vi "PicoStatus.vi"(1 "PICO STATUS":u32, 2 "error in":errorcluster, 3 "source":string) -> (0 "error out":errorcluster)   [LabVIEW 2016]
doc: "This VI checks the status value returned by calls to the driver. If the driver returns an error, the status member of the error cluster is set to 'true' and the error code and source are set."
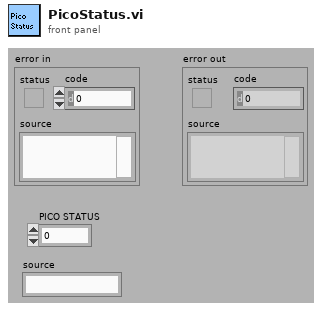
[diagram p1: front panel]
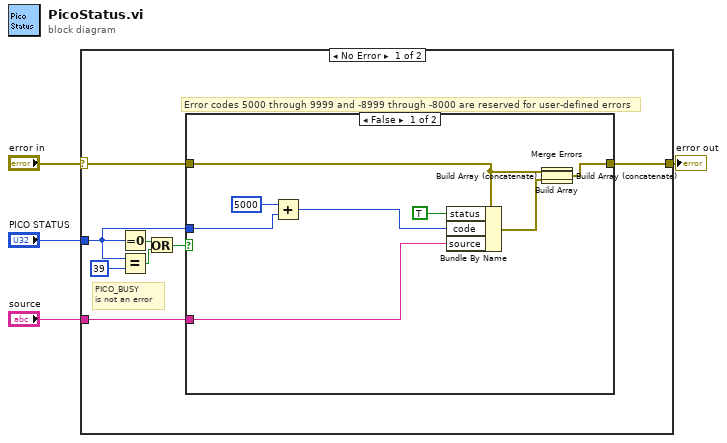
[diagram p0: block diagram]
diagram:
  n1 = case shown="No Error" "error in" {
    selector: "error in" -> [w11 w25]
    tunnel: [w12 w25] -> w4
    tunnel: "PICO STATUS" -> [w6 _]
    tunnel: "source" -> [w10 _]
    frame No Error {
      # "PICO_BUSY \nis not an error"
      # "Error codes 5000 through 9999 and -8999 through -8000 are reserved for user-defined errors"
      n2 = Equal To 0?(x=w6) -> (x = 0?=w9:bool)
      n3 = Equal?(x=w6, y=39) -> (x = y?=w7:bool)
      n4 = Or(x=w9, y=w7) -> (x .or. y?=w8:bool)
      n5 = case shown="False" w8 {
        tunnel: w11 -> [w22 w24]
        tunnel: [w23 w24] -> w12
        tunnel: w6 -> [w21 _]
        tunnel: w10 -> [w16 _]
        frame False {
          n6 = Add(x=5000, y=w21) -> (x+y=w17:u32)
          n7 = Bundle By Name(cluster=w22, "status"=TRUE, "code"=w17, "source"=w16) -> (w20:errorcluster)
          n8 = Build Array(w22, w20) -> (w15:errorcluster[])
          n9 = Build Array (concatenate)(w15) -> (w14:errorcluster[])
          n10 = Build Array (concatenate)(w14) -> (w13:errorcluster[])
          n11 = Merge Errors(w13) -> (w23:errorcluster)
        }
        frame True {
        }
      }
    }
    frame Error {
    }
  }
  "error out" <- w4
